vi "主程序.vi"() -> ()   [LabVIEW 2012]
panel:
  out "剩余旗子":u16
  out "剩余方块":u16
  out "游戏结果":bool
  in  "雷数":u16=20
  out "地图":dbl[][](array[numeric])
  out "雷区":dbl[][](array[numeric])
  out "start":bool
  out "簇":T1
  in  "列":u16=10
  in  "行":u16=10
  out "图片":picture
  # "目前配置：\n1608*872\n最大50列，27行"
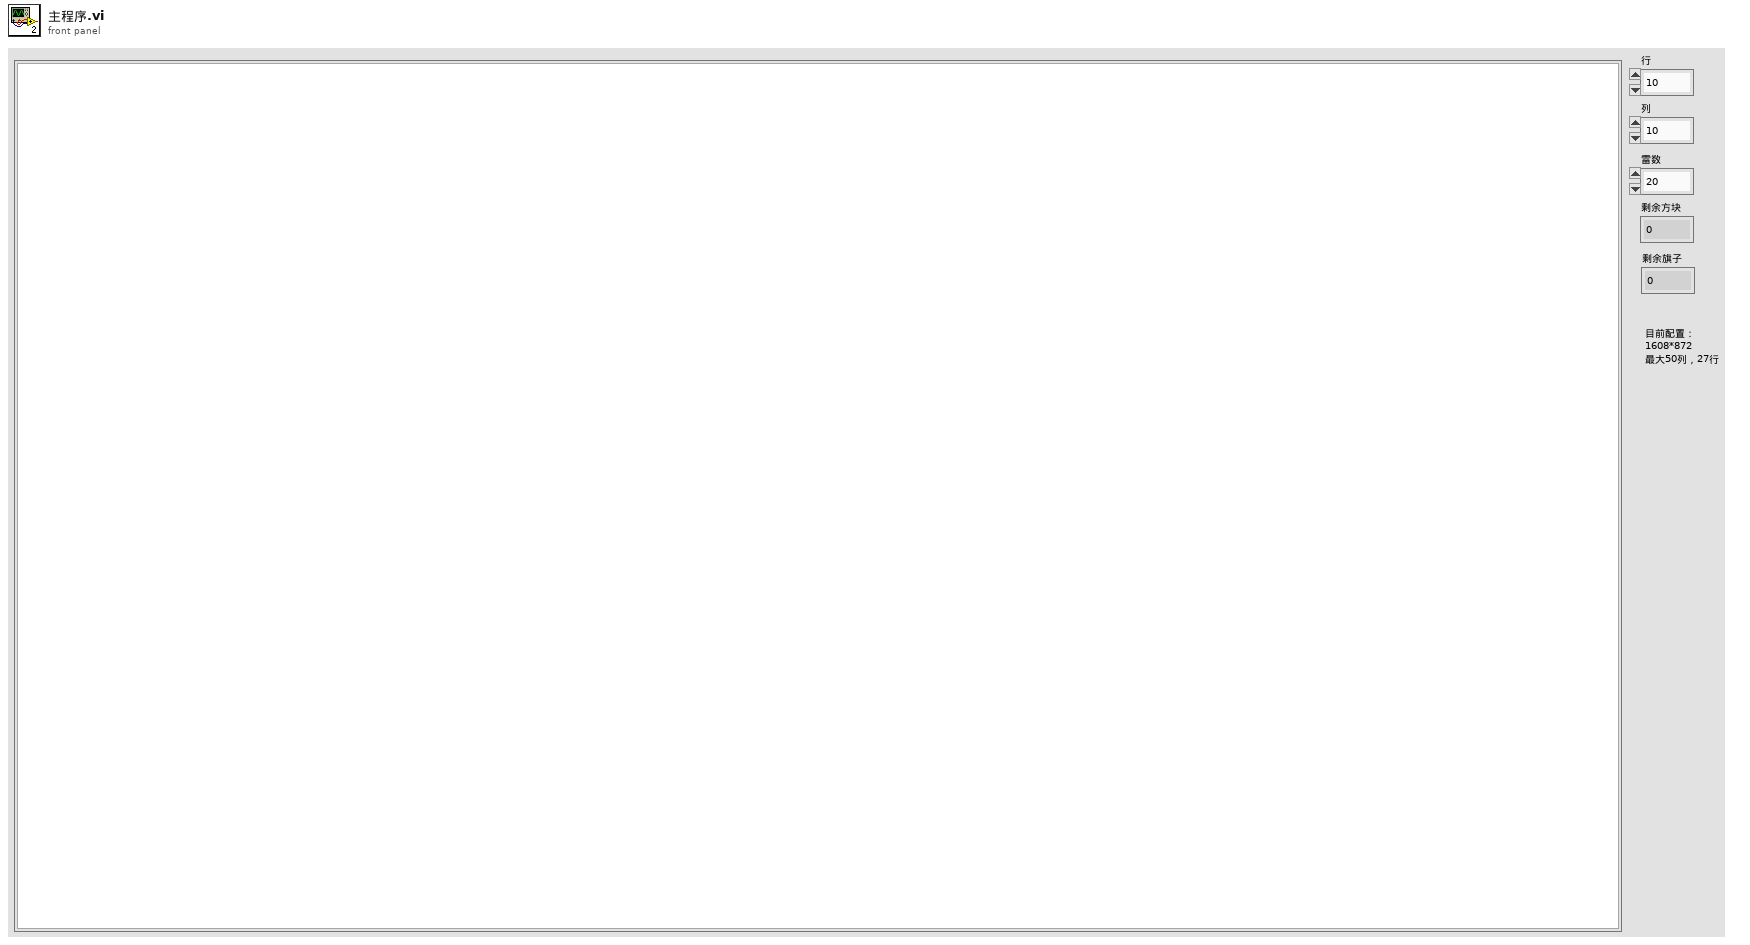
[diagram p1: front panel]
types:
  T1 = cluster{"数组":i32[][][], "colors":u32[], "mask":u8[]}
  T2 = typedef "LVPoint32TypeDef.ctl" = cluster{"Horizontal":i32, "Vertical":i32}
  T3 = typedef "LVPositionTypeDef.ctl" = cluster{"Left":i32, "Top":i32}
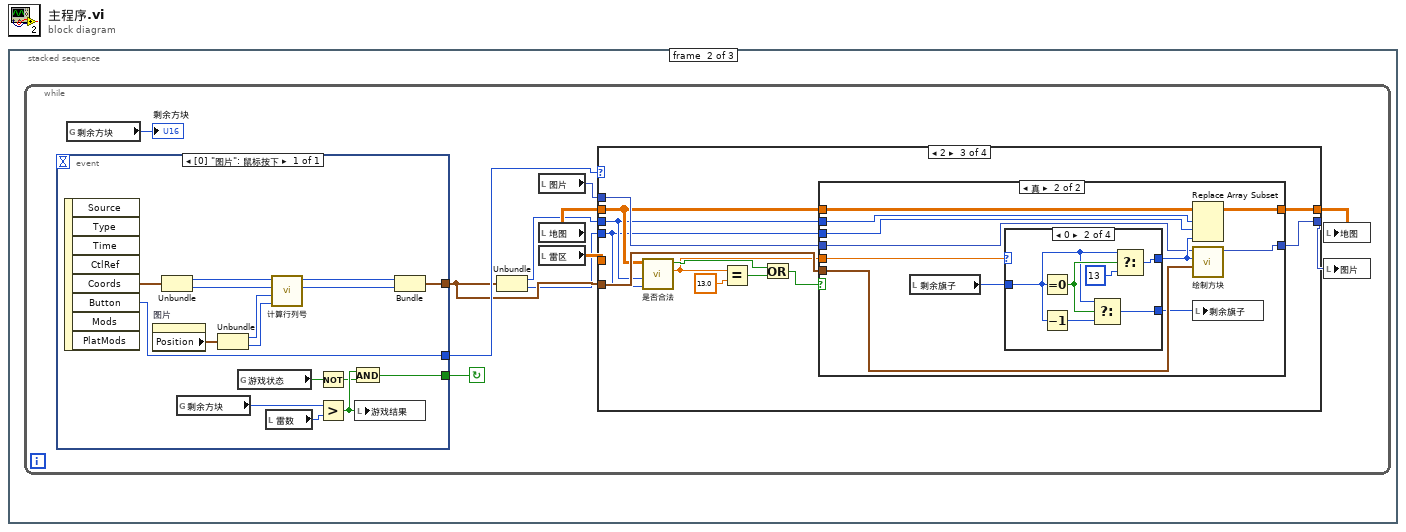
[diagram p0: block diagram]
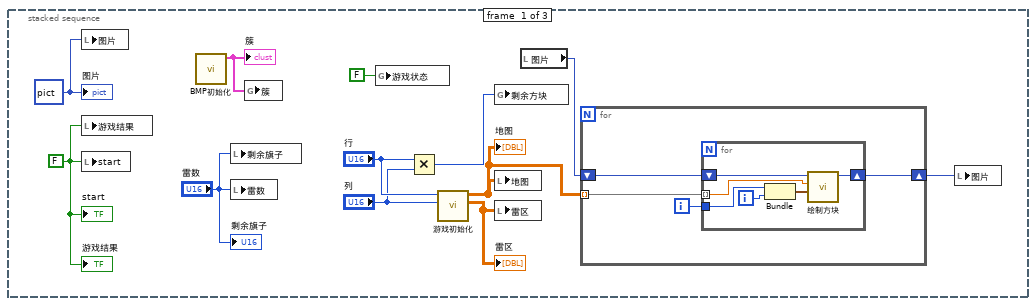
[diagram p2: hidden frame]
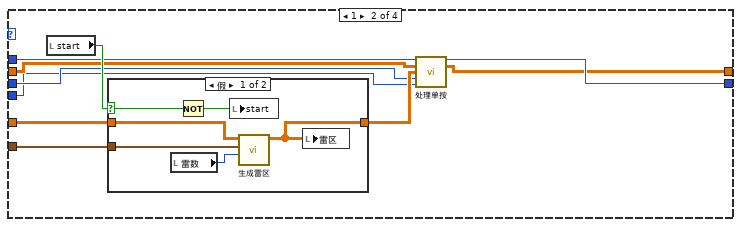
[diagram p4: hidden frame]
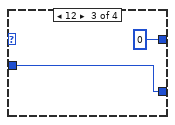
[diagram p8: hidden frame]
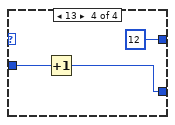
[diagram p9: hidden frame]
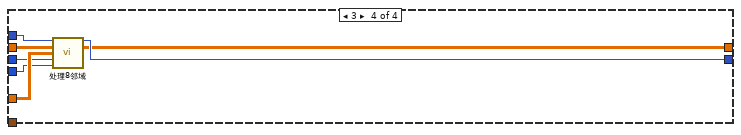
[diagram p10: hidden frame]
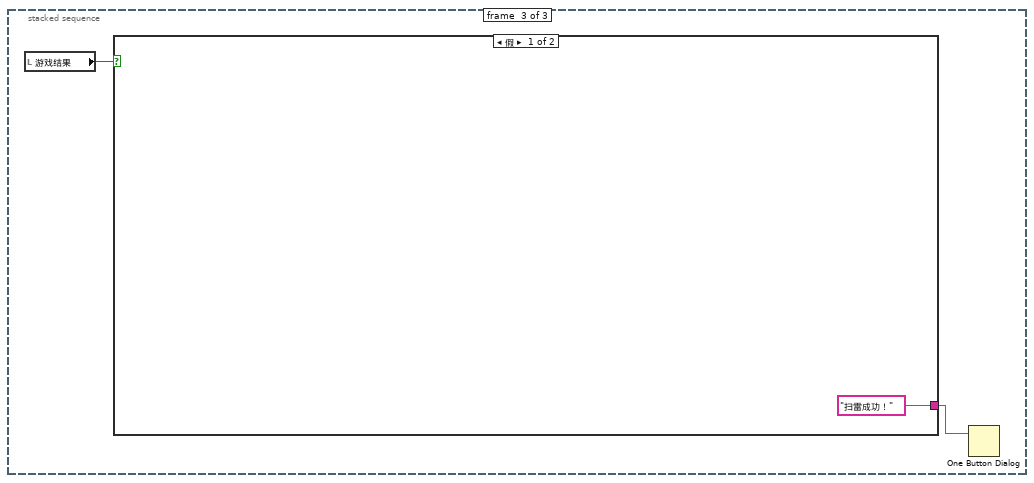
[diagram p11: hidden frame]
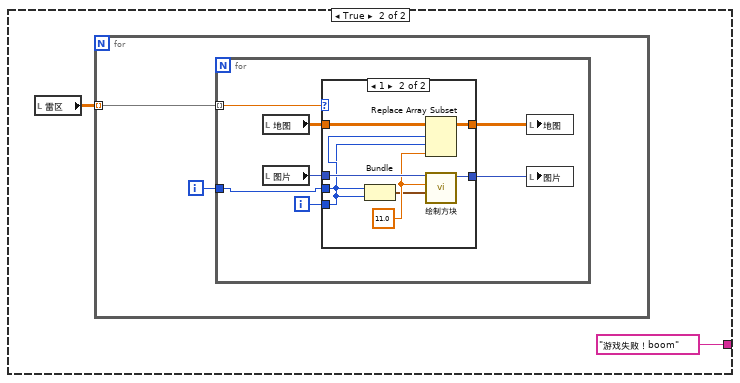
[diagram p12: hidden frame]
diagram:
  n1 = stacked-sequence {
    frame #0 {
      w5 = FALSE
      w3 = picture data[5B] ("原图片")
      n2 = local write "图片"(w3) -> ()
      n3 = local write "游戏结果"(w5) -> ()
      n4 = local write "start"(w5) -> ()
      n5 = call "BMP初始化.vi"() -> ("簇"=w8:T1)  [unwired: 11 in]
      "簇" <- w8
      n6 = local write "剩余旗子"("雷数") -> ()
      n7 = local write "雷数"("雷数") -> ()
      n8 = global write "全局变量.vi" "簇"(w8) -> ()
      n9 = global write "全局变量.vi" "游戏状态"(FALSE ("游戏状态")) -> ()
      n10 = Multiply(x="行", y="列") -> (x*y=w6:u16)
      n11 = call "游戏初始化.vi"("列数"="列", "行数"="行") -> ("雷区"=w12:dbl[][], "地图"=w11:dbl[][])  [unwired: 8 in]
      "雷区" <- w12
      "地图" <- w11
      n12 = global write "全局变量.vi" "剩余方块"(w6) -> ()
      n13 = local write "地图"(w11) -> ()
      n14 = local write "雷区"(w12) -> ()
      n15 = local read "图片"() -> (w10:picture)
      n16 = for {
        tunnel: w11 -> [w16] mode=indexing
        shift-right: [w13] -> w9
        shift-left: w10 -> [w14]
        i -> [w15]
        n17 = for {
          tunnel: w16 -> [w20] mode=indexing
          tunnel: w15 -> [w21]
          shift-right: [w17] -> w13
          shift-left: w14 -> [w18]
          i -> [w22]
          n18 = Bundle(w21, w22) -> (w19:cluster{i32, i32})  [unwired: 1 in]
          n19 = call "绘制方块.vi"("簇"=w19, "ID"=w20, "picture"=w18) -> ("new picture"=w17:picture)  [unwired: 8 in]
        }
      }
      n20 = local write "图片"(w9) -> ()
      "start" <- w5
      "图片" <- w3
      "游戏结果" <- w5
      "剩余旗子" <- "雷数"
    }
    frame #1 {
      n21 = while {
        stop <- w31 continue-if-true
        n22 = event shown="[0] \"图片\": 鼠标按下" {
          selector: _ -> [_]
          dyn-events: _ -> [_]
          timeout: _ -> [_]
          tunnel: [w112] -> w33
          tunnel: [w109] -> w32
          tunnel: [w105] -> w31
          event "图片": Mouse Down {
            n23 = event-data() -> ("Coords"=w113:T2, "Button"=w112:u16)  [unwired: 1 in, 6 out]
            n24 = property on="图片" class="Pict"() -> ("Position"=w100:T3)  [unwired: 2 in, 2 out]
            n25 = Unbundle(w113) -> ("Horizontal"=w102:i32, "Vertical"=w101:i32)
            n26 = global read "全局变量.vi" "剩余方块"() -> (w106:u16)
            n27 = Unbundle(w100) -> ("Left"=w99:i32, "Top"=w98:i32)
            n28 = global read "全局变量.vi" "游戏状态"() -> (w104:bool)
            n29 = local read "雷数"() -> (w107:u16)
            n30 = call "计算行列号.vi"("垂直偏移"=w98, "水平偏移"=w99, "垂直"=w101, "水平"=w102) -> ("列"=w110:i16, "行"=w111:i16)  [unwired: 6 in]
            n31 = Not(x=w104) -> (.not. x?=w103:bool)
            n32 = Greater?(x=w106, y=w107) -> (0:w108:bool)
            n33 = And(x=w108, y=w103) -> (x .and. y?=w105:bool)
            n34 = local write "游戏结果"(w108) -> ()
            n35 = Bundle("行"=w111, "列"=w110) -> (w109:cluster{"行":i16, "列":i16})  [unwired: 1 in]
          }
        }
        n36 = global read "全局变量.vi" "剩余方块"() -> (→"剩余方块":u16)
        n37 = Unbundle(w32) -> ("行"=w24:i16, "列"=w23:i16)
        n38 = local read "图片"() -> (w26:picture)
        n39 = local read "地图"() -> (w29:dbl[][])
        n40 = local read "雷区"() -> (w28:dbl[][])
        n41 = case shown="2" w33 {
          tunnel: w29 -> [w35 w39 w60 w96]
          tunnel: w28 -> [_ w44 _ w95]
          tunnel: w32 -> [_ w38 w63 _]
          tunnel: [w35 w40 w64 w91] -> w27
          tunnel: w26 -> [w34 w42 w61 w97]
          tunnel: [w34 w41 w62 w92] -> w25
          tunnel: w24 -> [_ w37 w59 w94]
          tunnel: w23 -> [_ w36 w58 w93]
          frame 0, Default {
          }
          frame 1 {
            n42 = local read "start"() -> (w45:bool)
            n43 = case shown="假" w45 {
              selector: w45 -> [w51 _]
              tunnel: w38 -> [w48 _]
              tunnel: w44 -> [w49 w52]
              tunnel: [w47 w52] -> w43
              frame False {
                n44 = local read "雷数"() -> (w46:u16)
                n45 = Not(x=w51) -> (.not. x?=w50:bool)
                n46 = local write "start"(w50) -> ()
                n47 = call "生成雷区.vi"("雷数"=w46, "firstPT"=w48, "输入"=w49) -> ("输出"=w47:dbl[][])  [unwired: 8 in]
                n48 = local write "雷区"(w47) -> ()
              }
              frame True {
              }
            }
            n49 = call "处理单按.vi"("图片"=w42, "地图"=w39, "雷区"=w43, "行"=w37, "列"=w36) -> ("图片 2"=w41:picture, "地图 2"=w40:dbl[][])  [unwired: 7 in, 2 out]
          }
          frame 2 {
            n50 = call "是否合法.vi"("列"=w58, "行"=w59, "地图"=w60) -> ("元素"=w53:dbl, "是否合法"=w55:bool)  [unwired: 7 in]
            n51 = Equal?(x=w53, y=13.0) -> (x = y?=w56:bool)
            n52 = Or(x=w55, y=w56) -> (x .or. y?=w54:bool)
            n53 = case shown="真" w54 {
              tunnel: [w65 w77] -> w64
              tunnel: w63 -> [_ w76]
              tunnel: [w66 w74] -> w62
              tunnel: w61 -> [w66 w73]
              tunnel: w60 -> [w65 w70]
              tunnel: w59 -> [_ w69]
              tunnel: w58 -> [_ w68]
              tunnel: w53 -> [_ w67]
              frame False {
              }
              frame True {
                n54 = local read "剩余旗子"() -> (w72:u16)
                n55 = case shown="0" w67 {
                  selector: w67 -> [w79 _ _ _]
                  tunnel: [w79 w80 0 12] -> w75
                  tunnel: w72 -> [w78 w81 w86 w89]
                  tunnel: [w78 w84 w86 w88] -> w71
                  frame -1, Default {
                  }
                  frame 0 {
                    n56 = Equal To 0?(x=w81) -> (x = 0?=w82:bool)
                    n57 = Decrement(x=w81) -> (x-1=w85:u16)
                    n58 = Select(t=w81, s=w82, f=w85) -> (s? t:f=w84:u16)
                    n59 = Select(t=w81, s=w82, f=13) -> (s? t:f=w80:i32)
                  }
                  frame 12 {
                  }
                  frame 13 {
                    n60 = Increment(x=w89) -> (x+1=w88:u16)
                  }
                }
                n61 = Replace Array Subset(array=w70, new element=w75, index (row)=w69, index (col)=w68) -> (w77:dbl[][])
                n62 = call "绘制方块.vi"("簇"=w76, "ID"=w75, "picture"=w73) -> ("new picture"=w74:picture)  [unwired: 8 in]
                n63 = local write "剩余旗子"(w71) -> ()
              }
            }
          }
          frame 3 {
            n64 = call "处理8邻域.vi"("图片"=w97, "地图"=w96, "雷区"=w95, "行"=w94, "列"=w93) -> ("图片 2"=w92:picture, "地图 2"=w91:dbl[][])  [unwired: 9 in]
          }
        }
        n65 = local write "地图"(w27) -> ()
        n66 = local write "图片"(w25) -> ()
      }
    }
    frame #2 {
      n67 = local read "游戏结果"() -> (w115:bool)
      n68 = case shown="假" w115 {
        tunnel: ["扫雷成功！" "游戏失败！boom"] -> w114
        frame False {
        }
        frame True {
          n69 = local read "雷区"() -> (w118:dbl[][])
          n70 = for {
            tunnel: w118 -> [w120] mode=indexing
            i -> [w119]
            n71 = for {
              tunnel: w120 -> [w127] mode=indexing
              tunnel: w119 -> [w125]
              i -> [w126]
              n72 = local read "地图"() -> (w121:dbl[][])
              n73 = local read "图片"() -> (w123:picture)
              n74 = case shown="1" w127 {
                tunnel: w126 -> [_ w131]
                tunnel: w125 -> [_ w132]
                tunnel: [w129 w134] -> w124
                tunnel: w123 -> [w129 w135]
                tunnel: [w128 w136] -> w122
                tunnel: w121 -> [w128 w137]
                frame 0, Default {
                }
                frame 1 {
                  w133 = 11.0 ("新元素/子数组")
                  n75 = Bundle(w132, w131) -> (w130:cluster{i32, i32})  [unwired: 1 in]
                  n76 = Replace Array Subset(array=w137, new element=w133, index (row)=w132, index (col)=w131) -> (w136:dbl[][])
                  n77 = call "绘制方块.vi"("簇"=w130, "ID"=w133, "picture"=w135) -> ("new picture"=w134:picture)  [unwired: 8 in]
                }
              }
              n78 = local write "地图"(w122) -> ()
              n79 = local write "图片"(w124) -> ()
            }
          }
        }
      }
      n80 = One Button Dialog(message=w114) -> ()  [unwired: 1 in, 1 out]
    }
  }
